vi "Get Metadata Paths.vi"(8 "error in (no error)":errorcluster, 11 "Device Model Str":string="myRIO") -> (0 "error out":errorcluster, 3 "Meta Data File Paths":path[](array[path]))   [LabVIEW 2021, in "Personality.lvlib"]
doc: "Gets the myRIO project meta dat file paths."
uses:
  <vilib>/myRIO/Common/FPGA Personality Framework/Personality.lvlib
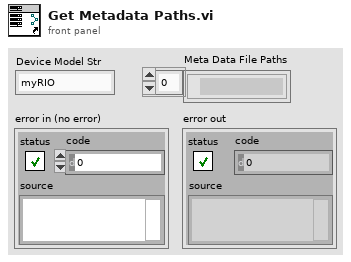
[diagram p1: front panel]
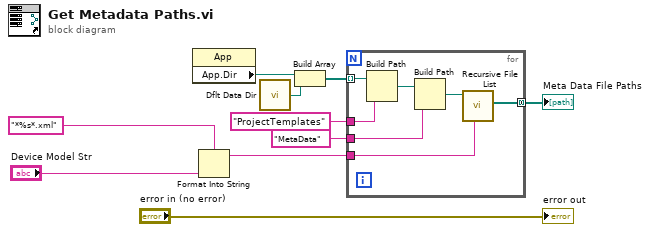
[diagram p0: block diagram]
diagram:
  n1 = property class="App"() -> ("App.Dir"=w9:path)  [unwired: 2 in, 2 out]
  n2 = Format Into String(format string="*%s*.xml", "Device Model Str") -> (resulting string=w2:string)  [unwired: 2 in, 1 out]
  n3 = call <vilib>:"Dflt Data Dir.vi"() -> ("App:Default Data Directory"=w10:path)
  n4 = Build Array(w9, w10) -> (w8:path[])
  n5 = for {
    tunnel: w8 -> [w17] mode=indexing
    tunnel: "ProjectTemplates" -> [w16]
    tunnel: "MetaData" -> [w14]
    tunnel: w2 -> [w13]
    tunnel: [w11] -> w4 mode=concatenating
    n6 = Build Path(base path=w17, name or relative path=w16) -> (appended path=w15:path)
    n7 = Build Path(base path=w15, name or relative path=w14) -> (appended path=w12:path)
    n8 = call <vilib>:"Recursive File List.vi"("pattern"=w13, "Folder Path"=w12) -> ("All Files in Dir"=w11:path[])  [unwired: 5 in, 4 out]
  }
  "Meta Data File Paths" <- w4
  "error out" <- "error in (no error)"
